vi "Stop Core.vi"(10 "final error code":i32, 11 "Command Processor in":refnum<class "Receiver Command.lvclass">) -> (3 "Command Processor out":refnum<class "Receiver Command.lvclass">)   [LabVIEW 2013, in "Receiver.lvlib" / "Receive Commands Using State Actors.lvlib" / "Receiver Command.lvclass"]
doc: "(<B>Filename</B>: Actor Framework.lvlib:Actor.lvclass:Stop Core.vi)\n\nDefines what the actor does before it stops. Use the <B>final error code</B> input to determine whether the actor shut down in response to an error.\n\nBy default, this method does nothing. A descendant class may override it to define behavior, such as shutting down any processes the actor initiated in its override of the Actor Core method."
uses:
  Receiver Command.lvclass
  Command/Command State Actor.lvclass
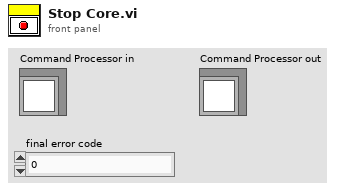
[diagram p1: front panel]
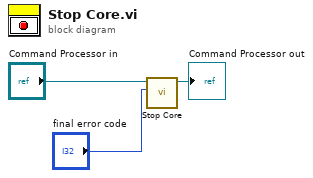
[diagram p0: block diagram]
diagram:
  n1 = call-parent "Stop Core.vi"("final error code"="final error code", "Command in"="Command Processor in") -> ("Command out"=→"Command Processor out":refnum<class "Receiver Command.lvclass">)  [unwired: 9 in]
